vi "Create String List.vi"(8 "error in (no error)":errorcluster, 11 "Initial Strings (empty list)":string[](array[string])) -> (0 "error out":errorcluster, 3 "StringList Reference":refnum<data-value>)   [LabVIEW 2015, in "StringList.lvlib" / "StringList.lvclass"]
uses:
  StringList.lvclass
  StringList.lvclass/StringList.ctl
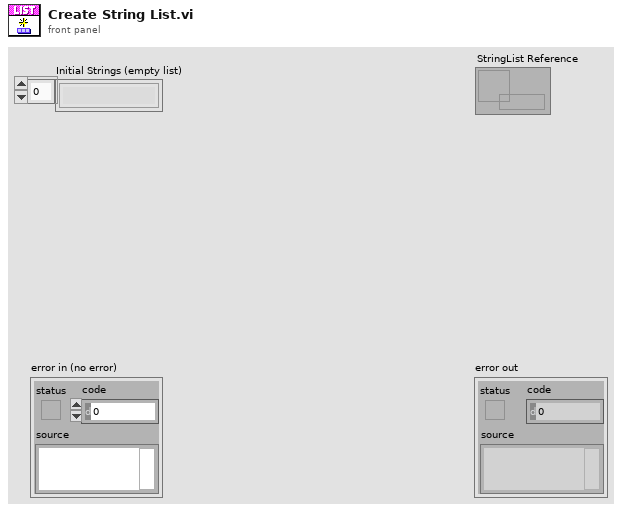
[diagram p1: front panel]
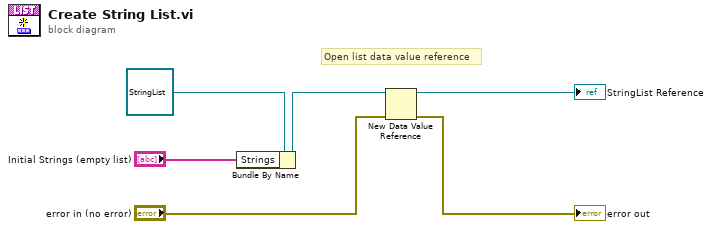
[diagram p0: block diagram]
diagram:
  # "Open list data value reference"
  n1 = Bundle By Name(cluster=refnum<class "StringList.lvclass"> refnum ("StringList in"), "Strings"="Initial Strings (empty list)") -> (w4:refnum<class "StringList.lvclass">)
  n2 = New Data Value Reference(data value=w4, error in="error in (no error)") -> (data value reference=→"StringList Reference":refnum<data-value>, error out=→"error out":errorcluster)
